vi "SubtractionClassTest.vi"(8 "error in (no error)":errorcluster) -> (0 "error out":errorcluster)   [LabVIEW 2023, in "TestLib.lvlib"]
doc: "This VI tests the subtract method class with some random test cases using caraya."
uses:
  Typedef/TestCaseSampleIO.ctl
  Arithmetic/Arithmetic.lvclass
  <vilib>/addons/_JKI Toolkits/Caraya/classes/Assert/Assert Equal Value_Variant.vi
  TestLib.lvlib
  <vilib>/addons/_JKI Toolkits/Caraya/classes/Test/Test.lvclass
  <vilib>/addons/_JKI Toolkits/Caraya/classes/Assert/Assert.lvclass
panel:
  # "SUBTRACTION CLASS TEST VI"
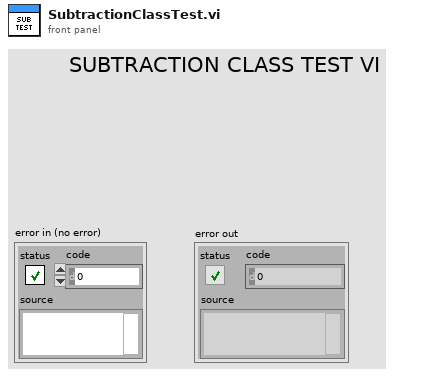
[diagram p1: front panel]
types:
  T1 = typedef "TestCaseSampleIO.ctl" = cluster{"Input1":dbl, "Input2":dbl, "Output":dbl}
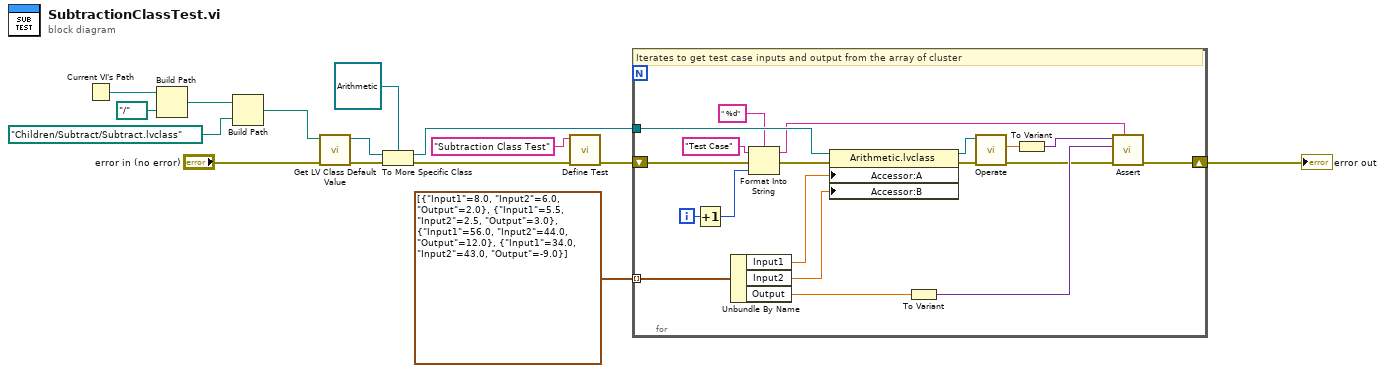
[diagram p0: block diagram]
diagram:
  n1 = Current VI's Path() -> (path=w11:path)
  n2 = Build Path(base path=w11, name or relative path=path "../..") -> (appended path=w9:path)
  n3 = Build Path(base path=w9, name or relative path=path "Children/Subtract/Subtract.lvclass") -> (appended path=w7:path)
  n4 = call <vilib>:"Get LV Class Default Value.vi"("error in (no error)"="error in (no error)", "class path"=w7) -> ("error out"=w2:errorcluster, "object"=w6:refnum<class>)  [unwired: 8 in]
  n5 = To More Specific Class(target class=refnum<class "Arithmetic.lvclass"> refnum ("Arithmetic.lvclass"), reference=w6, error in=w2) -> (specific class reference=w4:refnum<class "Arithmetic.lvclass">, error out=w1:errorcluster)
  n6 = call <vilib>:"Define Test.vi"("error in (no error)"=w1, "Label (VI Title)"="Subtraction Class Test") -> ("error out"=w15:errorcluster)  [unwired: 8 in, 1 out]
  n7 = for {
    tunnel: w4 -> [w34]
    shift-right: [w32] -> w13
    shift-left: w15 -> [w33]
    tunnel: T1[] [{"Input1"=8.0, "Input2"=6.0, "Output"=2.0}, {"Input1"=5.5, "Input2"=2.5, "Output"=3.0}, {"Input1"=56.0, "Input2"=44.0, "Output"=12.0}, {"Input1"=34.0, "Input2"=43.0, "Output"=-9.0}] -> [w31] mode=indexing
    i -> [w26]
    # "Iterates to get test case inputs and output from the array of cluster"
    n8 = Increment(x=w26) -> (x+1=w25:i32)
    n9 = Unbundle By Name(w31) -> ("Input1"=w30:dbl, "Input2"=w29:dbl, "Output"=w21:dbl)
    n10 = Format Into String(format string=" %d", initial string="Test Case", error in=w33, w25) -> (resulting string=w23:string, error out=w28:errorcluster)
    n11 = property class="Arithmetic.lvclass"(reference=w34, error in=w28, "Accessor:A"=w30, "Accessor:B"=w29) -> (reference out=w18:refnum<class "Arithmetic.lvclass">, error out=w19:errorcluster)
    n12 = To Variant(anything=w21) -> (Variant=w20:variant)
    n13 = call-dynamic "Operate.vi"("error in (no error)"=w19, "Arithmetic in"=w18) -> ("error out"=w17:errorcluster, "C"=w16:dbl)  [unwired: 7 in, 1 out]
    n14 = To Variant(anything=w16) -> (Variant=w22:variant)
    n15 = call-poly <vilib>:"Assert.vi"("Label"=w23, "error in (no error)"=w17, "Y"=w20, "X"=w22) -> ("error out"=w32:errorcluster)  [unwired: 6 in, 1 out]
  }
  "error out" <- w13
